vi "Teleop.vi"(0 "Call Context":T9) -> (6 "SubState 3":T4, 9 "SubState 4":T8, 11 "Loop 3 Data":T3, 14 "SubState 0":T4=enum."driver control", 15 "Loop 1 Data":T6, 16 "Loop 0 Data":T7, 17 "SubState 1":T4, 18 "Loop 2 Data":T5, 19 "SubState 2":T4)   [LabVIEW 2013]
uses:
  typedefs/State Machine/subStates.ctl
  <vilib>/Rock Robotics/WPI/DriverStation/WPI_DriverStationDerivedRobotMode.ctl
  typedefs/State Machine/singleUseSubstate.ctl
  typedefs/Loop Datatypes/Loop 0 Datatype.ctl
  typedefs/Loop Datatypes/Loop 1 Datatype.ctl
  typedefs/Loop Datatypes/Loop 2 Datatype.ctl
  typedefs/Loop Datatypes/Loop 3 Datatype.ctl
  <vilib>/Rock Robotics/WPI/Joystick/WPI_JoystickDevRef.ctl
  <vilib>/Rock Robotics/WPI/Joystick/WPI_JoystickDeviceEnum.ctl
  typedefs/fg_typedef.ctl
  typedefs/Vision/vision enable.ctl
  <vilib>/Rock Robotics/WPI/Joystick/WPI_JoystickGetSetRefNum.vi
panel:
  out "JS3":T1
  out "Drive to DC":bool
  out "JS1":T1
  out "JS2":T1
  out "Exit Value":i32=-1
  # "Loop Data and Substates"
  # "Drive Loop"
  # "State Machine Master Loop"
  # "Pickup/Passing Belts Loop"
  # "Pickup/Passing Arm Loop"
  # "Pneumatics Loop"
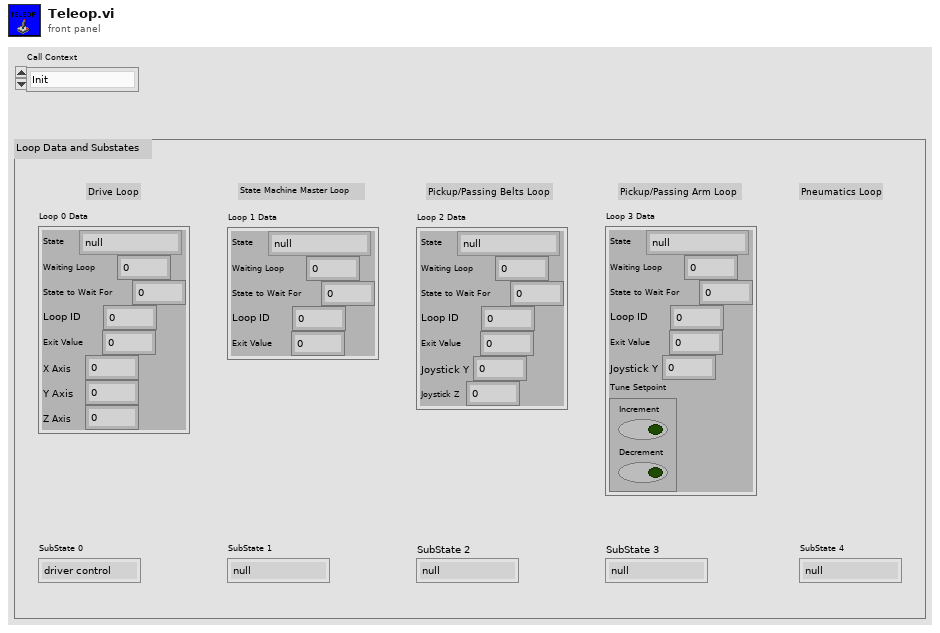
[diagram p1: front panel]
types:
  T1 = typedef "WPI_JoystickDevRef.ctl" = cluster{"Device":T2}
  T2 = typedef "WPI_JoystickDeviceEnum.ctl" = enum16{"USB 1", "USB 2", "USB 3", "USB 4", "Kinect 1", "Kinect 2"}
  T3 = typedef "Loop 3 Datatype.ctl" = cluster{"State":T4, "Waiting Loop":i32, "State to Wait For":i32, "Loop ID":i32, "Exit Value":i32, "Joystick Y":dbl, "Tune Setpoint":cluster{"Increment":bool, "Decrement":bool}}
  T4 = typedef "subStates.ctl" = enum16{"null", "wait", "driver control", "auto", "manual override", "hold position", "rotate", "pickup", "pass", "recover pass", "load", "goto shoot", "shoot high goal", "shoot low goal", "cancel arm", "cancel shooter", "end", "test"}
  T5 = typedef "Loop 2 Datatype.ctl" = cluster{"State":T4, "Waiting Loop":i32, "State to Wait For":i32, "Loop ID":i32, "Exit Value":i32, "Joystick Y":dbl, "Joystick Z":dbl}
  T6 = typedef "Loop 1 Datatype.ctl" = cluster{"State":T4, "Waiting Loop":i32, "State to Wait For":i32, "Loop ID":i32, "Exit Value":i32}
  T7 = typedef "Loop 0 Datatype.ctl" = cluster{"State":T4, "Waiting Loop":i32, "State to Wait For":i32, "Loop ID":i32, "Exit Value":i32, "X Axis":dbl, "Y Axis":dbl, "Z Axis":dbl}
  T8 = typedef "singleUseSubstate.ctl" = enum16{"null", "wait", "shift high", "shift low", "extend shooter", "retract shooter", "latch", "unlatch", "end"}
  T9 = typedef "WPI_DriverStationDerivedRobotMode.ctl" = enum16{"Init", "Execute", "Stop"}
  T10 = cluster{"axis 1 (x)":dbl, "axis 2 (y)":dbl, "axis 3 (throttle)":dbl, "axis 4":dbl, "axis 5":dbl, "axis 6":dbl}
  T11 = typedef "WPI_EncoderDevRef.ctl" = cluster{"DevStatus":errorcluster, "EncoderIndex":T12, "CounterIndex":T13, "DistancePerCount":dbl, "Decoding Type":T14}
  T12 = typedef "FPGA_EncoderIdx.ctl" = enum8{"Enc 0", "Enc 1", "Enc 2", "Enc 3", "Invalid"}
  T13 = typedef "FPGA_CounterCtrSystemIndex.ctl" = enum8{"Ctr 0", "Ctr 1", "Ctr 2", "Ctr 3", "Ctr 4", "Ctr 5", "Ctr 6", "Ctr 7", "Invalid"}
  T14 = typedef "WPI_EncoderType.ctl" = enum16{"1x", "2x", "4x"}
  T15 = typedef "vision enable.ctl" = enum16{"Enable", "Disable", "Stop"}
  T16 = typedef "fg_typedef.ctl" = enum16{"Get", "Set"}
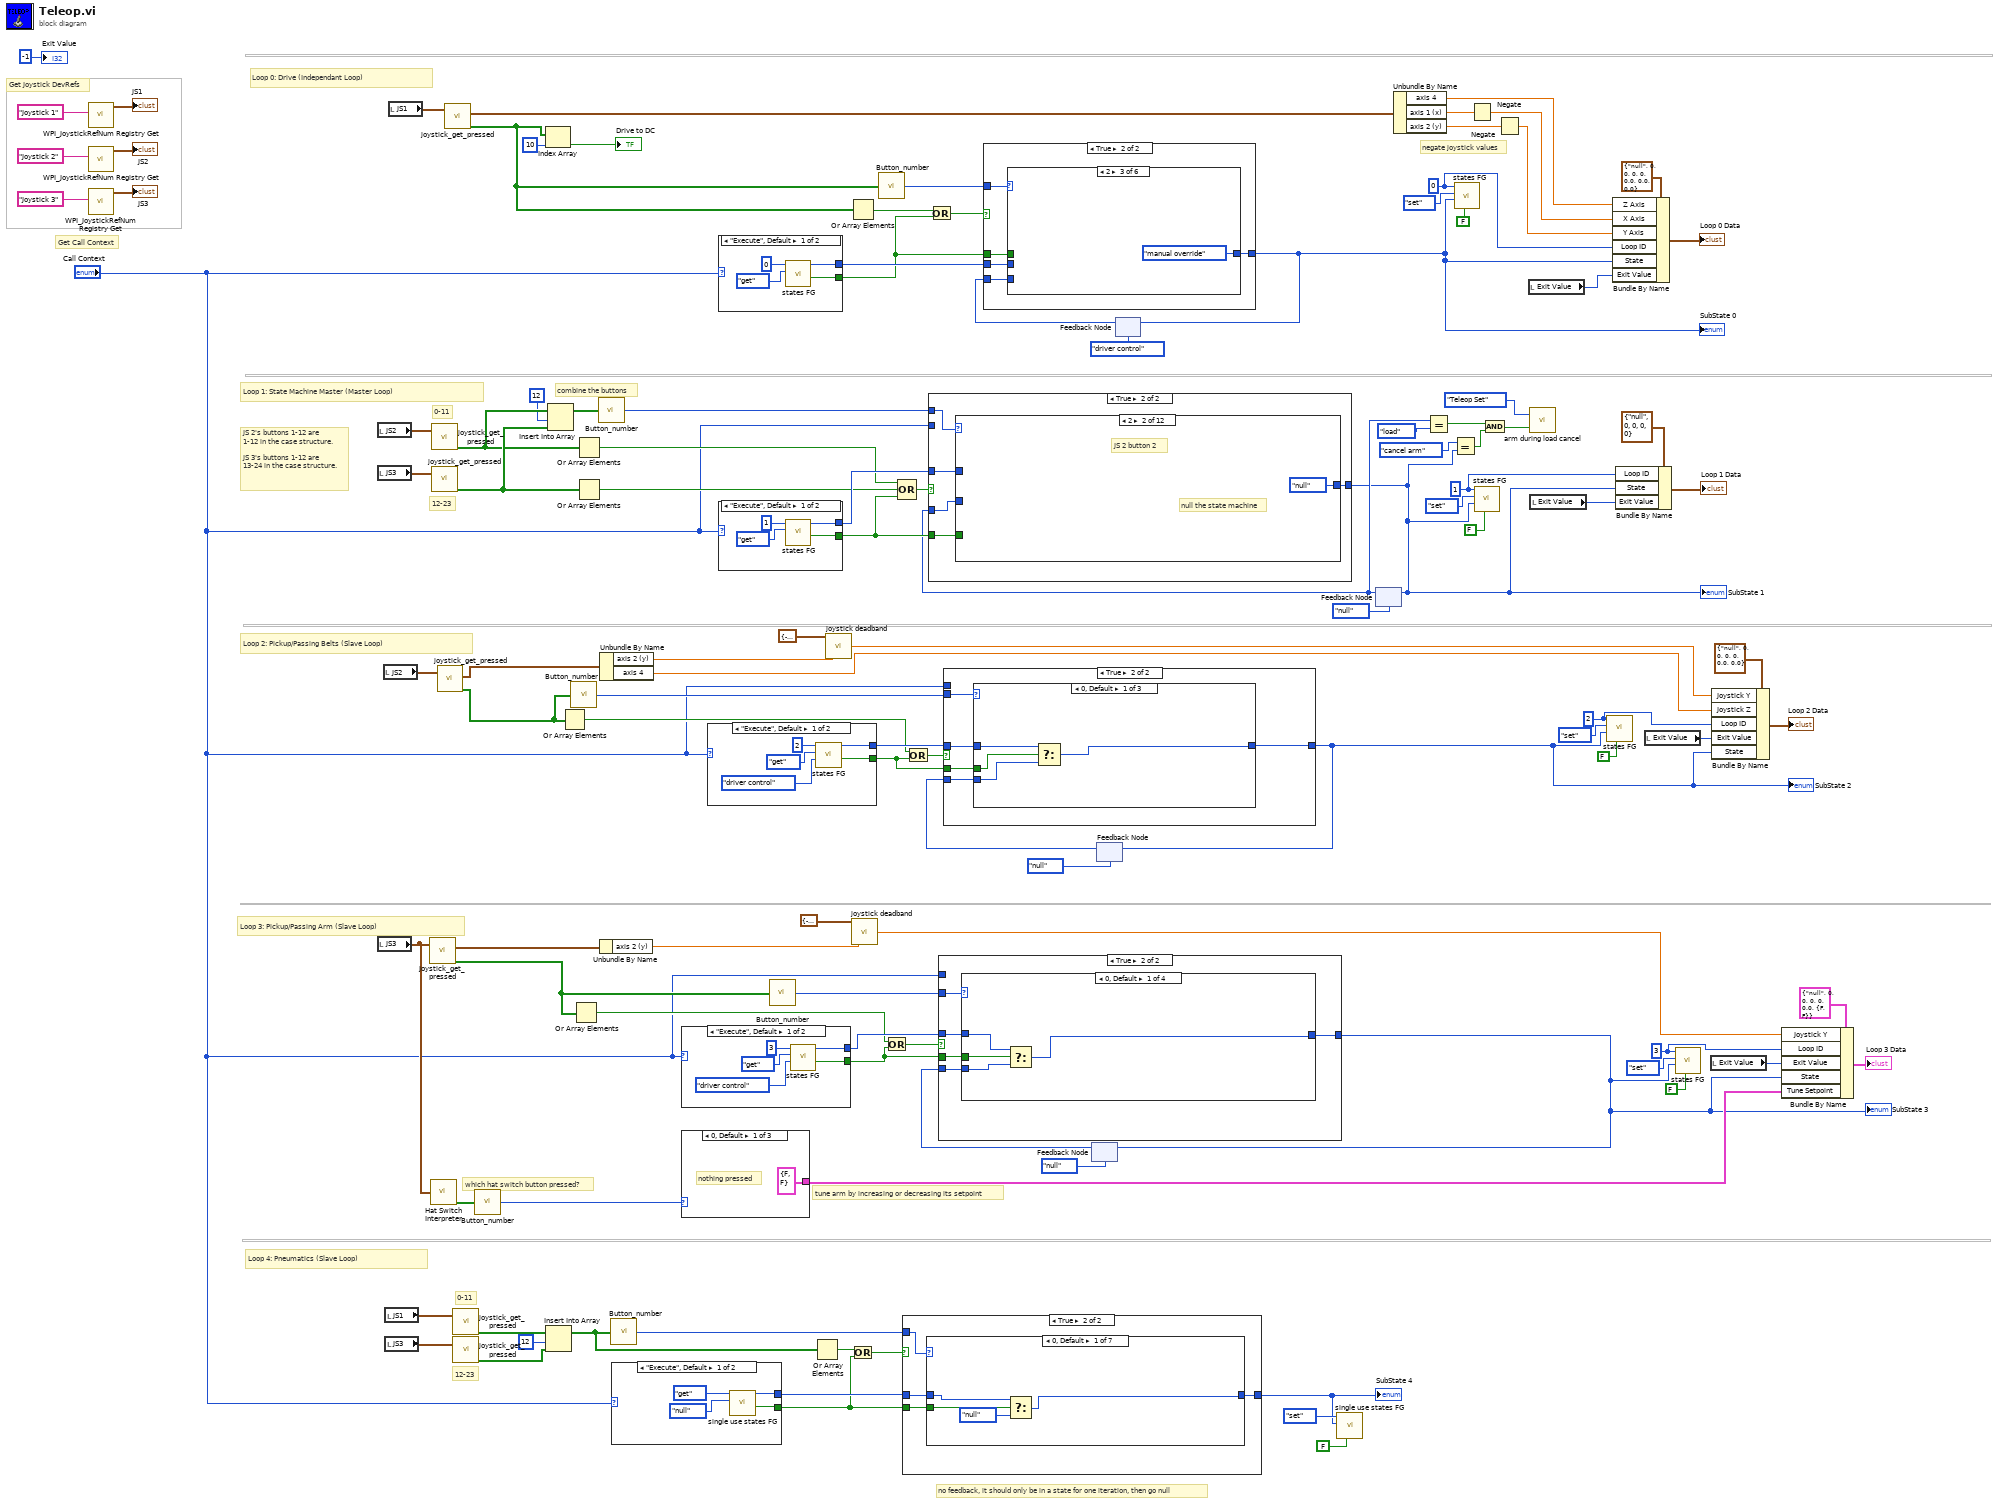
[diagram p0: block diagram]
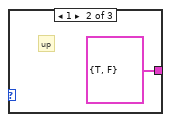
[diagram p2: hidden frame]
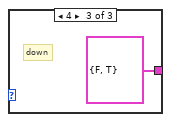
[diagram p3: hidden frame]
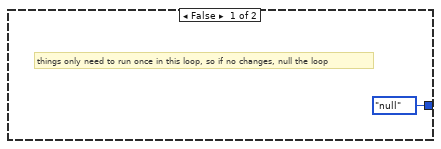
[diagram p4: hidden frame]
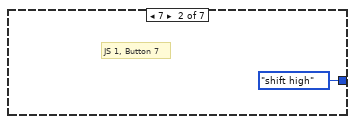
[diagram p5: hidden frame]
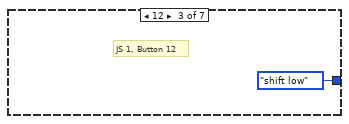
[diagram p6: hidden frame]
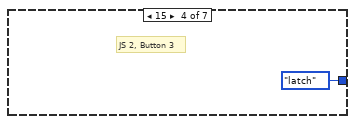
[diagram p7: hidden frame]
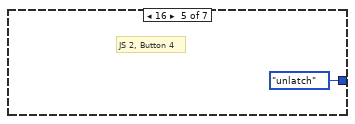
[diagram p8: hidden frame]
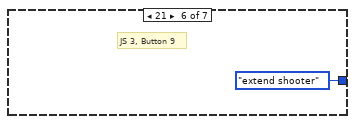
[diagram p9: hidden frame]
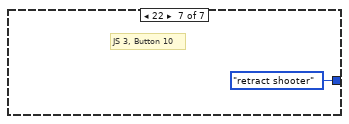
[diagram p10: hidden frame]
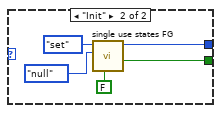
[diagram p11: hidden frame]
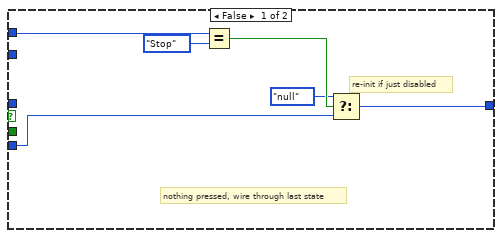
[diagram p12: hidden frame]
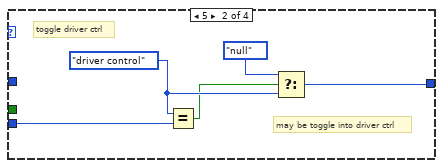
[diagram p13: hidden frame]
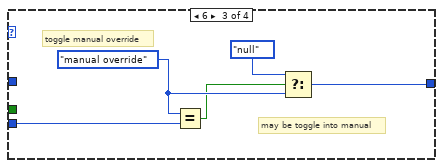
[diagram p14: hidden frame]
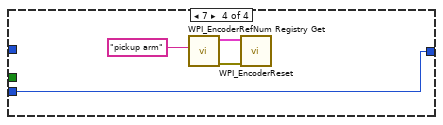
[diagram p15: hidden frame]
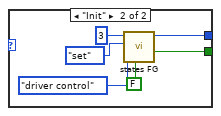
[diagram p16: hidden frame]
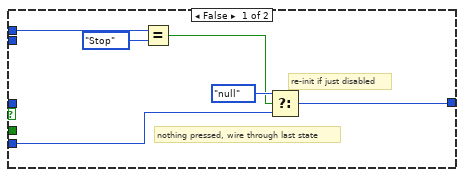
[diagram p17: hidden frame]
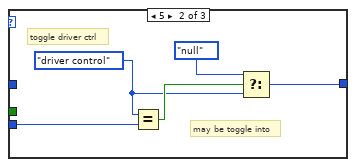
[diagram p18: hidden frame]
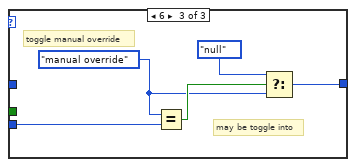
[diagram p19: hidden frame]
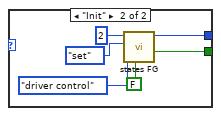
[diagram p20: hidden frame]
diagram:
  w90 = 3 ("Loop ID")
  w91 = 2 ("Loop ID")
  w100 = 1 ("Loop ID")
  w102 = 0 ("Loop ID")
  # "12-23"
  # "0-11"
  # "no feedback, it should only be in a state for one iteration, then go null"
  # "JS 2's buttons 1-12 are\n1-12 in the case structure.\n\nJS 3's buttons 1-12 are\n13-24 in the case structure."
  # "combine the buttons"
  # "12-23"
  # "0-11"
  # "tune arm by increasing or decreasing its setpoint"
  # "which hat switch button pressed?"
  # "negate joystick values"
  # "Get Call Context"
  # "Get Joystick DevRefs"
  # "Loop 3: Pickup/Passing Arm (Slave Loop)"
  # "Loop 4: Pneumatics (Slave Loop)"
  # "Loop 2: Pickup/Passing Belts (Slave Loop)"
  # "Loop 1: State Machine Master (Master Loop)"
  # "Loop 0: Drive (Independant Loop)"
  n1 = call <vilib>:"WPI_JoystickRefNum Registry Get.vi"("refnum name"="Joystick 1") -> ("JoystickDevRef"=→"JS1":T1)  [unwired: 9 in, 1 out]
  n2 = call <vilib>:"WPI_JoystickRefNum Registry Get.vi"("refnum name"="Joystick 2") -> ("JoystickDevRef"=→"JS2":T1)  [unwired: 9 in, 1 out]
  n3 = call <vilib>:"WPI_JoystickRefNum Registry Get.vi"("refnum name"="Joystick 3") -> ("JoystickDevRef"=→"JS3":T1)  [unwired: 9 in, 1 out]
  n4 = local read "JS2"() -> (w70:T1)
  n5 = local read "JS3"() -> (w26:T1)
  n6 = local read "JS3"() -> (w37:T1)
  n7 = local read "JS2"() -> (w48:T1)
  n8 = local read "JS1"() -> (w51:T1)
  n9 = local read "JS3"() -> (w11:T1)
  n10 = local read "JS1"() -> (w71:T1)
  n11 = call "joystick_get_pressed.vi"("JoystickDevRef 2"=w37) -> ("Axes"=w60:T10, "Buttons Pressed?"=w2:bool[])  [unwired: 1 in, 2 out]
  n12 = call "Hat Switch Interpreter.vi"("JoystickDevRef"=w37) -> ("Buttons"=w36:bool[])  [unwired: 4 out]
  n13 = call "joystick_get_pressed.vi"("JoystickDevRef 2"=w70) -> ("Buttons Pressed?"=w22:bool[])  [unwired: 1 in, 3 out]
  n14 = call "joystick_get_pressed.vi"("JoystickDevRef 2"=w26) -> ("Buttons Pressed?"=w23:bool[])  [unwired: 1 in, 3 out]
  n15 = call "joystick_get_pressed.vi"("JoystickDevRef 2"=w48) -> ("Axes"=w40:T10, "Buttons Pressed?"=w3:bool[])  [unwired: 1 in, 2 out]
  n16 = call "joystick_get_pressed.vi"("JoystickDevRef 2"=w71) -> ("Axes"=w75:T10, "Buttons Pressed?"=w53:bool[])  [unwired: 1 in, 2 out]
  n17 = call "joystick_get_pressed.vi"("JoystickDevRef 2"=w51) -> ("Buttons Pressed?"=w8:bool[])  [unwired: 1 in, 3 out]
  n18 = call "joystick_get_pressed.vi"("JoystickDevRef 2"=w11) -> ("Buttons Pressed?"=w9:bool[])  [unwired: 1 in, 3 out]
  n19 = call "Button_number.vi"("Button Array"=w36) -> ("Button Pressed"=w35:i32)
  n20 = Index Array(array=w53, index=10) -> (element=→"Drive to DC":bool)
  n21 = Insert Into Array(array=w8, index=12, new element=w9) -> (w7:bool[])
  n22 = Insert Into Array(array=w22, index=12, new element=w23) -> (w20:bool[])
  n23 = Or Array Elements(Boolean array=w3) -> (logical OR=w47:bool)
  n24 = call "Button_number.vi"("Button Array"=w3) -> ("Button Pressed"=w46:i32)
  n25 = Or Array Elements(Boolean array=w2) -> (logical OR=w59:bool)
  n26 = Or Array Elements(Boolean array=w22) -> (logical OR=w25:bool)
  n27 = Or Array Elements(Boolean array=w23) -> (logical OR=w24:bool)
  n28 = call "Button_number.vi"("Button Array"=w20) -> ("Button Pressed"=w64:i32)
  n29 = Unbundle By Name(w60) -> ("axis 2 (y)"=w56:dbl)
  n30 = Unbundle By Name(w40) -> ("axis 2 (y)"=w42:dbl, "axis 4"=w38:dbl)
  n31 = call "Button_number.vi"("Button Array"=w7) -> ("Button Pressed"=w28:i32)
  n32 = case shown="\"Execute\", Default" "Call Context" {
    tunnel: [w120 w123] -> w27
    tunnel: [w121 w122] -> w41
    frame "Execute", Default {
      n33 = call "single use states FG.vi"("substate"=singleUseSubstate."null" ("Enum"), "menu (get)"=enum16{"set", "get"}."get") -> ("exit out"=w120:bool, "substate out"=w121:T8)  [unwired: 6 in, 2 out]
    }
    frame "Init" {
      n34 = call "single use states FG.vi"("exit in"=FALSE, "substate"=singleUseSubstate."null", "menu (get)"=enum16{"set", "get"}."set") -> ("exit out"=w123:bool, "substate out"=w122:T8)  [unwired: 5 in, 2 out]
    }
  }
  n35 = case shown="\"Execute\", Default" "Call Context" {
    tunnel: [w129 w135] -> w57
    tunnel: [w127 w132] -> w88
    frame "Execute", Default {
      n36 = call "states FG.vi"("subState in"=subStates."driver control", "menu (get)"=enum16{"set", "get"}."get", "Loop ID"=3) -> ("exit out"=w129:bool, "subState out"=w127:T4)  [unwired: 5 in, 2 out]
    }
    frame "Init" {
      n37 = call "states FG.vi"("exit in"=FALSE, "subState in"=subStates."driver control", "menu (get)"=enum16{"set", "get"}."set", "Loop ID"=3) -> ("exit out"=w135:bool, "subState out"=w132:T4)  [unwired: 4 in, 2 out]
    }
  }
  n38 = case shown="0, Default" w35 {
    tunnel: [cluster{"Increment":bool, "Decrement":bool} {"Increment"=FALSE, "Decrement"=FALSE} cluster{"Increment":bool, "Decrement":bool} {"Increment"=TRUE, "Decrement"=FALSE} cluster{"Increment":bool, "Decrement":bool} {"Increment"=FALSE, "Decrement"=TRUE}] -> w33
    frame 0, Default {
      # "nothing pressed"
    }
    frame 1 {
      # "up"
    }
    frame 4 {
      # "down"
    }
  }
  n39 = case shown="\"Execute\", Default" "Call Context" {
    tunnel: [w143 w149] -> w62
    tunnel: [w141 w146] -> w106
    frame "Execute", Default {
      n40 = call "states FG.vi"("subState in"=subStates."driver control", "menu (get)"=enum16{"set", "get"}."get", "Loop ID"=2) -> ("exit out"=w143:bool, "subState out"=w141:T4)  [unwired: 5 in, 2 out]
    }
    frame "Init" {
      n41 = call "states FG.vi"("exit in"=FALSE, "subState in"=subStates."driver control", "menu (get)"=enum16{"set", "get"}."set", "Loop ID"=2) -> ("exit out"=w149:bool, "subState out"=w146:T4)  [unwired: 4 in, 2 out]
    }
  }
  n42 = case shown="\"Execute\", Default" "Call Context" {
    tunnel: [w153 w158] -> w68
    tunnel: [w152 w156] -> w105
    frame "Execute", Default {
      n43 = call "states FG.vi"("menu (get)"=enum16{"set", "get"}."get", "Loop ID"=0) -> ("exit out"=w153:bool, "subState out"=w152:T4)  [unwired: 6 in, 2 out]
    }
    frame "Init" {
      n44 = call "states FG.vi"("exit in"=FALSE, "menu (get)"=enum16{"set", "get"}."set", "Loop ID"=0) -> ("exit out"=w158:bool, "subState out"=w156:T4)  [unwired: 5 in, 2 out]
    }
  }
  n45 = case shown="\"Execute\", Default" "Call Context" {
    tunnel: [w162 w167] -> w65
    tunnel: [w161 w165] -> w104
    frame "Execute", Default {
      n46 = call "states FG.vi"("menu (get)"=enum16{"set", "get"}."get", "Loop ID"=1) -> ("exit out"=w162:bool, "subState out"=w161:T4)  [unwired: 6 in, 2 out]
    }
    frame "Init" {
      n47 = call "states FG.vi"("exit in"=FALSE, "menu (get)"=enum16{"set", "get"}."set", "Loop ID"=1) -> ("exit out"=w167:bool, "subState out"=w165:T4)  [unwired: 5 in, 2 out]
    }
  }
  n48 = call "Button_number.vi"("Button Array"=w2) -> ("Button Pressed"=w58:i32)
  n49 = Or Array Elements(Boolean array=w7) -> (logical OR=w29:bool)
  n50 = call "joystick deadband.vi"("Joystick In"=w42, "Deadband Range"=cluster{"Deadband Min":dbl, "Deadband Max":dbl} {"Deadband Min"=-0.09, "Deadband Max"=0.09}) -> ("Joystick Out"=w39:dbl)  [unwired: 4 in]
  n51 = Or Array Elements(Boolean array=w53) -> (logical OR=w69:bool)
  n52 = Or(x=w29, y=w27) -> (x .or. y?=w30:bool)
  n53 = call "joystick deadband.vi"("Joystick In"=w56, "Deadband Range"=cluster{"Deadband Min":dbl, "Deadband Max":dbl} {"Deadband Min"=-0.09, "Deadband Max"=0.09}) -> ("Joystick Out"=w34:dbl)  [unwired: 4 in]
  n54 = call "Button_number.vi"("Button Array"=w53) -> ("Button Pressed"=w74:i32)
  n55 = Or(x=w59, y=w57) -> (x .or. y?=w61:bool)
  n56 = Compound Arithmetic op=OR(w25, w24, w65) -> (w66:bool)
  n57 = case shown="True" w30 {
    tunnel: [singleUseSubstate."null" ("Enum") w171] -> w5
    tunnel: w41 -> [_ w172]
    tunnel: w28 -> [_ w173]
    tunnel: w27 -> [_ w174]
    frame False {
      # "things only need to run once in this loop, so if no changes, null the loop"
    }
    frame True {
      n58 = case shown="0, Default" w173 {
        tunnel: w174 -> [w178 _ _ _ _ _ _]
        tunnel: w172 -> [w177 _ _ _ _ _ _]
        tunnel: [w176 singleUseSubstate."shift high" ("Enum") singleUseSubstate."shift low" ("Enum") singleUseSubstate."latch" ("Enum") singleUseSubstate."unlatch" ("Enum") singleUseSubstate."extend shooter" ("Enum") singleUseSubstate."retract shooter" ("Enum")] -> w171
        frame 0, Default {
          n59 = Select(t=w177, s=w178, f=singleUseSubstate."null") -> (s? t:f=w176:T8)
        }
        frame 7 {
          # "JS 1, Button 7"
        }
        frame 12 {
          # "JS 1, Button 12"
        }
        frame 15 {
          # "JS 2, Button 3"
        }
        frame 16 {
          # "JS 2, Button 4"
        }
        frame 21 {
          # "JS 3, Button 9"
        }
        frame 22 {
          # "JS 3, Button 10"
        }
      }
    }
  }
  "SubState 4" <- w5
  n60 = Or(x=w47, y=w62) -> (x .or. y?=w63:bool)
  n61 = Or(x=w69, y=w68) -> (x .or. y?=w67:bool)
  n62 = feedback #1(subStates."null" ("Drive SubState")) -> (w85:T4)
  n63 = case shown="True" w61 {
    tunnel: w85 -> [w187 w191]
    tunnel: [w186 w192] -> w32
    tunnel: w88 -> [_ w193]
    tunnel: w58 -> [_ w195]
    tunnel: w57 -> [_ w194]
    tunnel: "Call Context" -> [w185 _]
    frame False {
      # "nothing pressed, wire through last state"
      # "re-init if just disabled"
      n64 = Equal?(x=w185, y=WPI_DriverStationDerivedRobotMode."Stop") -> (x = y?=w189:bool)
      n65 = Select(t=subStates."null", s=w189, f=w187) -> (s? t:f=w186:T4)
    }
    frame True {
      n66 = case shown="0, Default" w195 {
        tunnel: w194 -> [w199 _ _ _]
        tunnel: w191 -> [w198 w200 w205 w213]
        tunnel: w193 -> [w197 _ _ _]
        tunnel: [w196 w201 w206 w213] -> w192
        frame 0, Default {
          n67 = Select(t=w197, s=w199, f=w198) -> (s? t:f=w196:T4)
        }
        frame 5 {
          w203 = subStates."driver control" ("Drive SubState")
          # "may be toggle into driver ctrl"
          # "toggle driver ctrl"
          n68 = Equal?(x=w203, y=w200) -> (x = y?=w202:bool)
          n69 = Select(t=subStates."null", s=w202, f=w203) -> (s? t:f=w201:T4)
        }
        frame 6 {
          w209 = subStates."manual override" ("Drive SubState")
          # "may be toggle into manual"
          # "toggle manual override"
          n70 = Equal?(x=w209, y=w205) -> (x = y?=w207:bool)
          n71 = Select(t=subStates."null", s=w207, f=w209) -> (s? t:f=w206:T4)
        }
        frame 7 {
          n72 = call <vilib>:"WPI_EncoderRefNum Registry Get.vi"("refnum name"="pickup arm") -> ("error out"=w211:errorcluster, "EncoderDevRef"=w210:T11)  [unwired: 9 in]
          n73 = call <vilib>:"WPI_EncoderReset.vi"("error in (no error)"=w211, "EncoderDevRef"=w210) -> ()  [unwired: 8 in, 2 out]
        }
      }
    }
  }
  "SubState 3" <- w32
  n74 = feedback-in #1(w32) -> ()
  n75 = feedback #2(subStates."null" ("Drive SubState")) -> (w109:T4)
  n76 = case shown="True" w63 {
    tunnel: w109 -> [w215 w221]
    tunnel: [w214 w220] -> w31
    tunnel: w106 -> [_ w222]
    tunnel: w46 -> [_ w224]
    tunnel: w62 -> [_ w223]
    tunnel: "Call Context" -> [w216 _]
    frame False {
      # "re-init if just disabled"
      # "nothing pressed, wire through last state"
      n77 = Equal?(x=w216, y=WPI_DriverStationDerivedRobotMode."Stop") -> (x = y?=w218:bool)
      n78 = Select(t=subStates."null", s=w218, f=w215) -> (s? t:f=w214:T4)
    }
    frame True {
      n79 = case shown="0, Default" w224 {
        tunnel: w223 -> [w228 _ _]
        tunnel: w222 -> [w227 _ _]
        tunnel: w221 -> [w226 w233 w235]
        tunnel: [w225 w229 w234] -> w220
        frame 0, Default {
          n80 = Select(t=w227, s=w228, f=w226) -> (s? t:f=w225:T4)
        }
        frame 5 {
          w231 = subStates."driver control" ("Drive SubState")
          # "may be toggle into"
          # "toggle driver ctrl"
          n81 = Equal?(x=w231, y=w233) -> (x = y?=w232:bool)
          n82 = Select(t=subStates."null", s=w232, f=w231) -> (s? t:f=w229:T4)
        }
        frame 6 {
          w236 = subStates."manual override" ("Drive SubState")
          # "may be toggle into"
          # "toggle manual override"
          n83 = Equal?(x=w236, y=w235) -> (x = y?=w238:bool)
          n84 = Select(t=subStates."null", s=w238, f=w236) -> (s? t:f=w234:T4)
        }
      }
    }
  }
  "SubState 2" <- w31
  n85 = feedback-in #2(w31) -> ()
  n86 = feedback #3(subStates."driver control" ("Drive SubState")) -> (w111:T4)
  n87 = case shown="True" w67 {
    tunnel: w111 -> [w239 w241]
    tunnel: [w239 w240] -> w50
    tunnel: w105 -> [_ w242]
    tunnel: w74 -> [_ w244]
    tunnel: w68 -> [_ w243]
    frame False {
      # "keep current state, no change necessary"
    }
    frame True {
      n88 = case shown="2" w244 {
        tunnel: w243 -> [w248 _ _ _ _ _]
        tunnel: w242 -> [w247 _ _ _ _ _]
        tunnel: w241 -> [w246 w253 _ w255 w263 _]
        tunnel: [w245 w249 subStates."manual override" ("Drive SubState") w255 w264 subStates."driver control" ("Drive SubState")] -> w240
        frame 0, Default {
          n89 = Select(t=w247, s=w248, f=w246) -> (s? t:f=w245:T4)
        }
        frame 1 {
          w250 = subStates."hold position" ("x")
          # "button 1, hold position toggle"
          n90 = Equal?(x=w250, y=w253) -> (x = y?=w252:bool)
          n91 = Select(t=subStates."driver control" ("Drive SubState"), s=w252, f=w250) -> (s? t:f=w249:T4)
        }
        frame 2 {
        }
        frame 8 {
          n92 = disable-structure shown="Enabled" {
            frame Enabled {
              w258 = vision_enable."Enable" ("y")
              # "toggle vision"
              n93 = call "vision_fg.vi"("Menu"=fg_typedef."Get") -> ("State Out"=w260:T15)  [unwired: 2 in, 1 out]
              n94 = Equal?(x=w260, y=w258) -> (x = y?=w259:bool)
              n95 = Select(t=vision_enable."Disable" ("y"), s=w259, f=w258) -> (s? t:f=w256:T15)
              n96 = call "vision_fg.vi"("Action"=w256, "Menu"=fg_typedef."Set") -> ()  [unwired: 1 in, 2 out]
            }
            frame Disabled {
              # "no vision in teleop"
            }
          }
        }
        frame 10 {
          n97 = disable-structure shown="Enabled" {
            disable-tunnel: [subStates."goto shoot" ("Drive SubState") w268] -> w264
            disable-tunnel: w263 -> [_ w268]
            frame Disabled {
              # "go to shoot location"
              n98 = call "vision_fg.vi"("Action"=vision_enable."Enable", "Menu"=fg_typedef."Set") -> ()  [unwired: 1 in, 2 out]
            }
            frame Enabled {
            }
          }
        }
        frame 11 {
          # "put robot drive in driver control"
          n99 = call "vision_fg.vi"("Action"=vision_enable."Disable", "Menu"=fg_typedef."Set") -> ()  [unwired: 1 in, 2 out]
        }
      }
    }
  }
  "SubState 0" <- w50
  n100 = feedback-in #3(w50) -> ()
  n101 = call "single use states FG.vi"("exit in"=FALSE, "substate"=w5, "menu (get)"=enum16{"set", "get"}."set") -> ()  [unwired: 5 in, 4 out]
  n102 = feedback #4(subStates."null" ("Drive SubState")) -> (w17:T4)
  n103 = case shown="True" w66 {
    tunnel: w17 -> [w274 w281]
    tunnel: [w272 w280] -> w14
    tunnel: w104 -> [_ w282]
    tunnel: w64 -> [_ w279]
    tunnel: w65 -> [_ w278]
    tunnel: "Call Context" -> [w277 _]
    frame False {
      # "re-init if just disabled"
      # "nothing pressed here, move along (wire through the previous state)"
      n104 = Equal?(x=w277, y=WPI_DriverStationDerivedRobotMode."Stop") -> (x = y?=w275:bool)
      n105 = Select(t=subStates."null", s=w275, f=w274) -> (s? t:f=w272:T4)
    }
    frame True {
      n106 = case shown="2" w279 {
        tunnel: w282 -> [w286 _ _ _ _ _ _ _ _ _ _ _]
        tunnel: w281 -> [w285 _ _ _ _ _ _ _ _ _ _ _]
        tunnel: [w284 subStates."null" ("Drive SubState") subStates."load" ("Drive SubState") subStates."cancel arm" ("Drive SubState") subStates."recover pass" ("Drive SubState") subStates."pickup" ("Drive SubState") subStates."pass" ("Drive SubState") subStates."shoot high goal" ("Drive SubState") subStates."load" ("Drive SubState") subStates."manual override" ("Drive SubState") subStates."shoot low goal" ("Drive SubState") subStates."cancel shooter" ("Drive SubState")] -> w280
        tunnel: w278 -> [w283 _ _ _ _ _ _ _ _ _ _ _]
        frame 0, Default {
          n107 = Select(t=w286, s=w283, f=w285) -> (s? t:f=w284:T4)
        }
        frame 2 {
          # "null the state machine"
          # "JS 2 button 2"
        }
        frame 8 {
          w288 = fg_typedef."Set" ("Menu")
          # "button 8, JS 2"
          n108 = call "safe shoot error.vi"("Can Shoot Safely?"=FALSE, "Menu"=w288) -> ()  [unwired: 1 out]
          n109 = call "load mode fg.vi"("Load Mode"=enum16{"Feild Load", "Human Player Load"}."Human Player Load", "Menu"=w288) -> ()  [unwired: 1 out]
        }
        frame 9 {
          # "button 9, JS 2"
        }
        frame 10 {
          # "button 10, JS2, recover pass"
        }
        frame 11 {
          # "button 11, JS 2"
        }
        frame 12 {
          # "button 12, JS 2"
        }
        frame 13 {
          # "button 1, JS 3"
        }
        frame 14 {
          w298 = fg_typedef."Set" ("Menu")
          # "button 2, JS 3"
          n110 = call "safe shoot error.vi"("Can Shoot Safely?"=FALSE, "Menu"=w298) -> ()  [unwired: 1 out]
          n111 = call "load mode fg.vi"("Load Mode"=enum16{"Feild Load", "Human Player Load"}."Feild Load", "Menu"=w298) -> ()  [unwired: 1 out]
        }
        frame 20 {
          # "manual shoot"
          # "button 8, JS 3"
        }
        frame 23 {
          # "button 11, JS 3"
        }
        frame 24 {
          # "button 12, JS 3"
        }
      }
    }
  }
  "SubState 1" <- w14
  n112 = feedback-in #4(w14) -> ()
  n113 = Unbundle By Name(w75) -> ("axis 4"=w54:dbl, "axis 1 (x)"=w79:dbl, "axis 2 (y)"=w78:dbl)
  n114 = Equal?(x=w17, y=subStates."load") -> (x = y?=w15:bool)
  n115 = Equal?(x=subStates."cancel arm" ("y"), y=w14) -> (x = y?=w16:bool)
  n116 = call "states FG.vi"("exit in"=FALSE, "subState in"=w50, "menu (get)"=enum16{"set", "get"}."set", "Loop ID"=w102) -> ()  [unwired: 4 in, 4 out]
  n117 = Negate(x=w79) -> (-x=w77:dbl)
  n118 = call "states FG.vi"("exit in"=FALSE, "subState in"=w14, "menu (get)"=enum16{"set", "get"}."set", "Loop ID"=w100) -> ()  [unwired: 4 in, 4 out]
  n119 = And(x=w15, y=w16) -> (x .and. y?=w13:bool)
  n120 = Negate(x=w78) -> (-x=w76:dbl)
  n121 = local read "Exit Value"() -> (w98:i32)
  n122 = call "arm during load cancel.vi"("Arm Canceled During Load?"=w13, "Mode"=enum16{"Get", "Set", "Teleop Set"}."Teleop Set") -> ()  [unwired: 1 out]
  n123 = local read "Exit Value"() -> (w97:i32)
  n124 = call "states FG.vi"("exit in"=FALSE, "subState in"=w31, "menu (get)"=enum16{"set", "get"}."set", "Loop ID"=w91) -> ()  [unwired: 4 in, 4 out]
  n125 = Bundle By Name(cluster=T7 {"State"=enum."null", "Waiting Loop"=0, "State to Wait For"=0, "Loop ID"=0, "Exit Value"=0, "X Axis"=0.0, "Y Axis"=0.0, "Z Axis"=0.0} ("Cluster"), "Z Axis"=w54, "X Axis"=w77, "Y Axis"=w76, "Loop ID"=w102, "State"=w50, "Exit Value"=w98) -> (→"Loop 0 Data":T7)
  n126 = Bundle By Name(cluster=T6 {"State"=enum."null", "Waiting Loop"=0, "State to Wait For"=0, "Loop ID"=0, "Exit Value"=0} ("Cluster"), "Loop ID"=w100, "State"=w14, "Exit Value"=w97) -> (→"Loop 1 Data":T6)
  n127 = local read "Exit Value"() -> (w92:i32)
  n128 = call "states FG.vi"("exit in"=FALSE, "subState in"=w32, "menu (get)"=enum16{"set", "get"}."set", "Loop ID"=w90) -> ()  [unwired: 4 in, 4 out]
  n129 = local read "Exit Value"() -> (w89:i32)
  n130 = Bundle By Name(cluster=T5 {"State"=enum."null", "Waiting Loop"=0, "State to Wait For"=0, "Loop ID"=0, "Exit Value"=0, "Joystick Y"=0.0, "Joystick Z"=0.0} ("Loop 2 Data"), "Joystick Y"=w39, "Joystick Z"=w38, "Loop ID"=w91, "Exit Value"=w92, "State"=w31) -> (→"Loop 2 Data":T5)
  n131 = Bundle By Name(cluster=T3 {"State"=enum."null", "Waiting Loop"=0, "State to Wait For"=0, "Loop ID"=0, "Exit Value"=0, "Joystick Y"=0.0, "Tune Setpoint"={"Increment"=FALSE, "Decrement"=FALSE}} ("Loop 3 Data"), "Joystick Y"=w34, "Loop ID"=w90, "Exit Value"=w89, "State"=w32, "Tune Setpoint"=w33) -> (→"Loop 3 Data":T3)
  "Exit Value" <- -1 ("Exit Value")
